vi "Renishaw-XL80_GetAutoCompensationMode.vi"(8 "error in (no error)":errorcluster, 11 "Renishaw-XL80_EMU in":refnum<class "Renishaw-XL80_EMU.lvclass">) -> (0 "error out":errorcluster, 2 "AutoCompensationMode":i32(ring) items=["AUTO_COMPENSATION_OFF"=0, "AUTO_COMPENSATION_AIR"=1, "AUTO_COMPENSATION_FULL"=3], 3 "Renishaw-XL80_EMU out":refnum<class "Renishaw-XL80_EMU.lvclass">)   [LabVIEW 2024, in "Renishaw-XL80_EMU.lvclass"]
doc: "Reading this property retrieves the current compensation mode.\n\nDefinition\nHRESULT\nget_AutoCompensationMode(\n [out, retval] AUTO_COMPENSATION_MODES* pVal\n);\nParameters\npVal\nA variable that will be set to one of the values in the enumerated type AUTO_COMPENSATION_MODES.\n\nComments\nReading this property will always retrieve the current compensation mode.\n\nThe property will normally return an HRESULT of S_OK. However, it will return E_POINTER if the client supplies a null pointer for pVal."
uses:
  Renishaw-XL80_EMU.lvclass
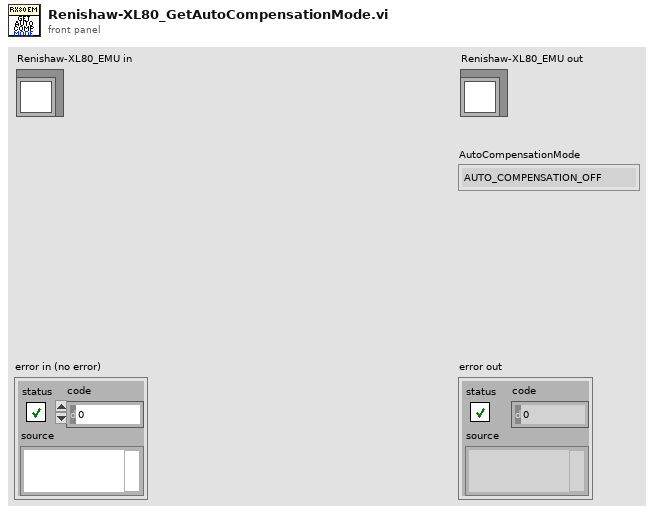
[diagram p1: front panel]
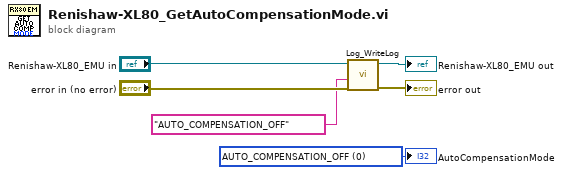
[diagram p0: block diagram]
diagram:
  w6 = 0 items=["AUTO_COMPENSATION_OFF"=0, "AUTO_COMPENSATION_AIR"=1, "AUTO_COMPENSATION_FULL"=3] ("AutoCompensationMode")
  n1 = call-dynamic "Log_WriteLog.vi"("error in (no error)"="error in (no error)", "Response"="AUTO_COMPENSATION_OFF", "Log in"="Renishaw-XL80_EMU in") -> ("error out"=→"error out":errorcluster, "Log out"=→"Renishaw-XL80_EMU out":refnum<class "Renishaw-XL80_EMU.lvclass">)  [unwired: 7 in]
  "AutoCompensationMode" <- w6
